vi "uService SV (Un)Deploy.vi"(6 "Undeploy?":bool, 8 "error in (no error)":errorcluster, 11 "uService Template in":refnum<class "Father of all uServices.lvclass">) -> (0 "error out":errorcluster, 3 "uService Template out":refnum<class "Father of all uServices.lvclass">)   [LabVIEW 2020, in "TALOS.lvlib" / "Father of all uServices.lvlib" / "Father of all uServices.lvclass"]
uses:
  Father of all uServices.lvclass
  <vilib>/AdvancedString/Delimited String to 1D String Array.vi
  <vilib>/Utility/LVClass/Get LV Class Name.vi
  Support VIs/Global Memory.vi
  TALOS.lvlib
  Classes/Circus Shared Variables/Circus Shared Variables.lvclass
panel:
  out "Library path":path
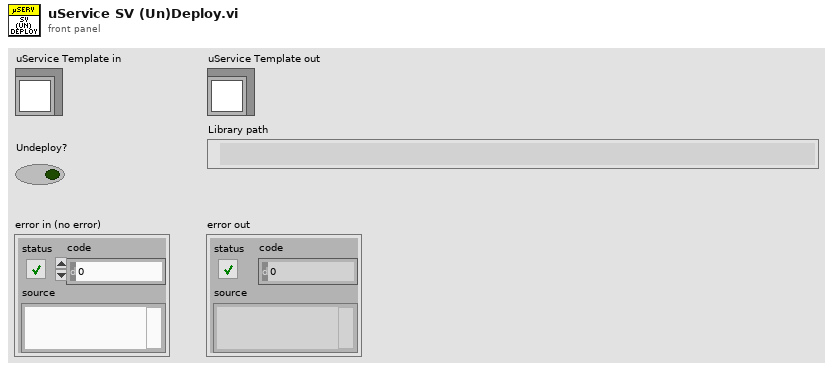
[diagram p1: front panel]
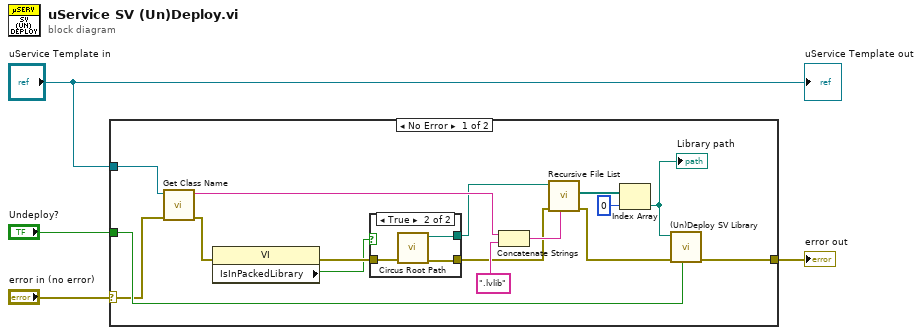
[diagram p0: block diagram]
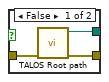
[diagram p2: hidden frame]
diagram:
  n1 = case shown="No Error" "error in (no error)" {
    selector: "error in (no error)" -> [w13 w27]
    tunnel: "Undeploy?" -> [w17 _]
    tunnel: [w16 w27] -> w3
    tunnel: "uService Template in" -> [w12 _]
    frame No Error {
      n2 = call "Get Class Name.vi"("error in (no error)"=w13, "object"=w12) -> ("error out"=w14:errorcluster, "Class Name"=w15:string)  [unwired: 8 in]
      n3 = property on="Property Node" class="VI"(error in=w14) -> (error out=w20:errorcluster, "IsInPackedLibrary"=w18:bool)  [unwired: 1 in, 1 out]
      n4 = case shown="True" w18 {
        tunnel: w20 -> [w23 w26]
        tunnel: [w22 w25] -> w6
        tunnel: [w21 w24] -> w11
        frame False {
          n5 = call "TALOS Root path.vi"("error in (no error)"=w23) -> ("error out"=w22:errorcluster, "TALOS Root Path"=w21:path)  [unwired: 9 in]
        }
        frame True {
          n6 = call "Circus Root Path.vi"("error in (no error)"=w26) -> ("error out"=w25:errorcluster, "Circus Root Path"=w24:path)  [unwired: 9 in]
        }
      }
      n7 = Concatenate Strings(w15, ".lvlib" ("string")) -> (w10:string)
      n8 = call <vilib>:"Recursive File List.vi"("pattern"=w10, "error in (no error)"=w6, "Folder Path"=w11) -> ("error out"=w5:errorcluster, "All Files in Dir"=w9:path[])  [unwired: 4 in, 3 out]
      n9 = Index Array(array=w9, index=0) -> (element=w7:path)
      "Library path" <- w7
      n10 = call "(Un)Deploy SV Library.vi"("Undeploy?"=w17, "error in (no error)"=w5, "Library path"=w7) -> ("error out"=w16:errorcluster)  [unwired: 8 in]
    }
    frame Error {
    }
  }
  "error out" <- w3
  "uService Template out" <- "uService Template in"
